vi "SubVI PhaseSpace.vi"() -> ()   [LabVIEW 2011]
uses:
  NCML-PhaseSpace/ctrOWLMarker.ctl
  ctlSeqFNs_SubVI PhaseSpace.ctl
  ctlPkgPhaseSpace.ctl
  ctlSeqFNs_SubVI ATI.ctl
  ctlTrialState.ctl
  ctlSeqFNs.ctl
  NCML-PhaseSpace/ctrCommonFlags.ctl
  NCML-PhaseSpace/ctrSetsFlags.ctl
  GLOBAL -MAIN.vi
  C:/Program Files/Phasespace/libowlsock.dll
panel:
  out "Hz":dbl(graph)
  out "save file":path
  in  "Read Cycle Time (s)":dbl=0.05 min=0.01 max=10.0 step=0.01 format="%.2f"
  out "recording?":bool
  out "markers obtained (err: <0)":u16
  out "markers":T1[](array[typedef])
  in  "marker count":i32=16
  out "connected?":bool
  in  "server IP":string="192.168.0.101"
  in  "STOP":bool
  # "Parallel SubVI PhaseSpace"
  # "Acquires PhaseSpace data and Trigger signal\nSaves TDMS file."
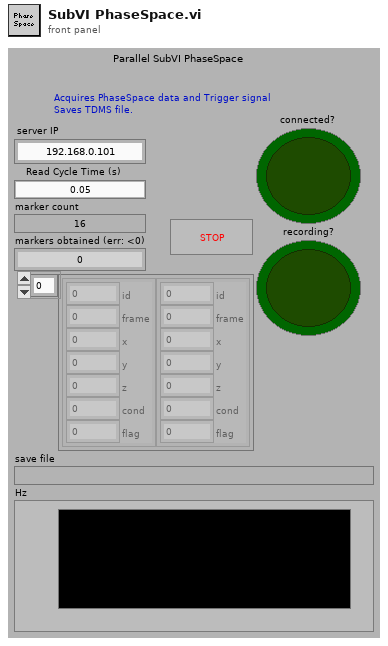
[diagram p1: front panel]
types:
  T1 = typedef "ctrOWLMarker.ctl" = cluster{"id":i32, "frame":i32, "x":sgl, "y":sgl, "z":sgl, "cond":sgl, "flag":u32}
  T2 = typedef "ctlPkgPhaseSpace.ctl" = cluster{"VIRef":refnum<vi>, "PhaseSpace":refnum<k34>, "PhaseSpace Ch names":string[], "Markers":T1[], "Markers Ch count":i32, "tick ini":i64, "ATI":refnum<queue>, "Trigger events":T3, "connected to server?":bool, "recording?":bool, "MAIN":refnum<queue>, "tick pre":i64, "Markers count":u16}
  T3 = typedef "ctlTrialState.ctl" = enum16{"no events", "ready", "start", "hold", "stop", "end"}
  T4 = typedef "ctlSeqFNs_SubVI PhaseSpace.ctl" = enum16{"INITIALIZE", "IDLE", "READY", "SEND2MAIN", "TRIGGER", "END", "ERROR", "EXIT"}
  T5 = typedef "ctlSeqFNs.ctl" = enum16{"INITIALIZE MAIN", "UpdateProtocol", "INITIALIZE Sub", "IDLE", "Ready", "Events", "Get PhaseSpace", "Get ATI", "Finish", "End PhaseSpace", "End ATI", "ERROR", "EXIT"}
  T6 = typedef "ctlSeqFNs_SubVI ATI.ctl" = enum16{"INITIALIZE", "IDLE", "READY", "SEND2MAIN", "CALIB Load", "BIAS", "TRIGGER", "END", "ERROR", "EXIT"}
  T7 = enum16{"ALIGN -CENTER", "ALIGN -TOP LEFT", "ALIGN -AS IS", "ALIGN -CUSTOM"}
  T8 = typedef "ctrCommonFlags.ctl" = u16
  T9 = typedef "ctrSetsFlags.ctl" = u16
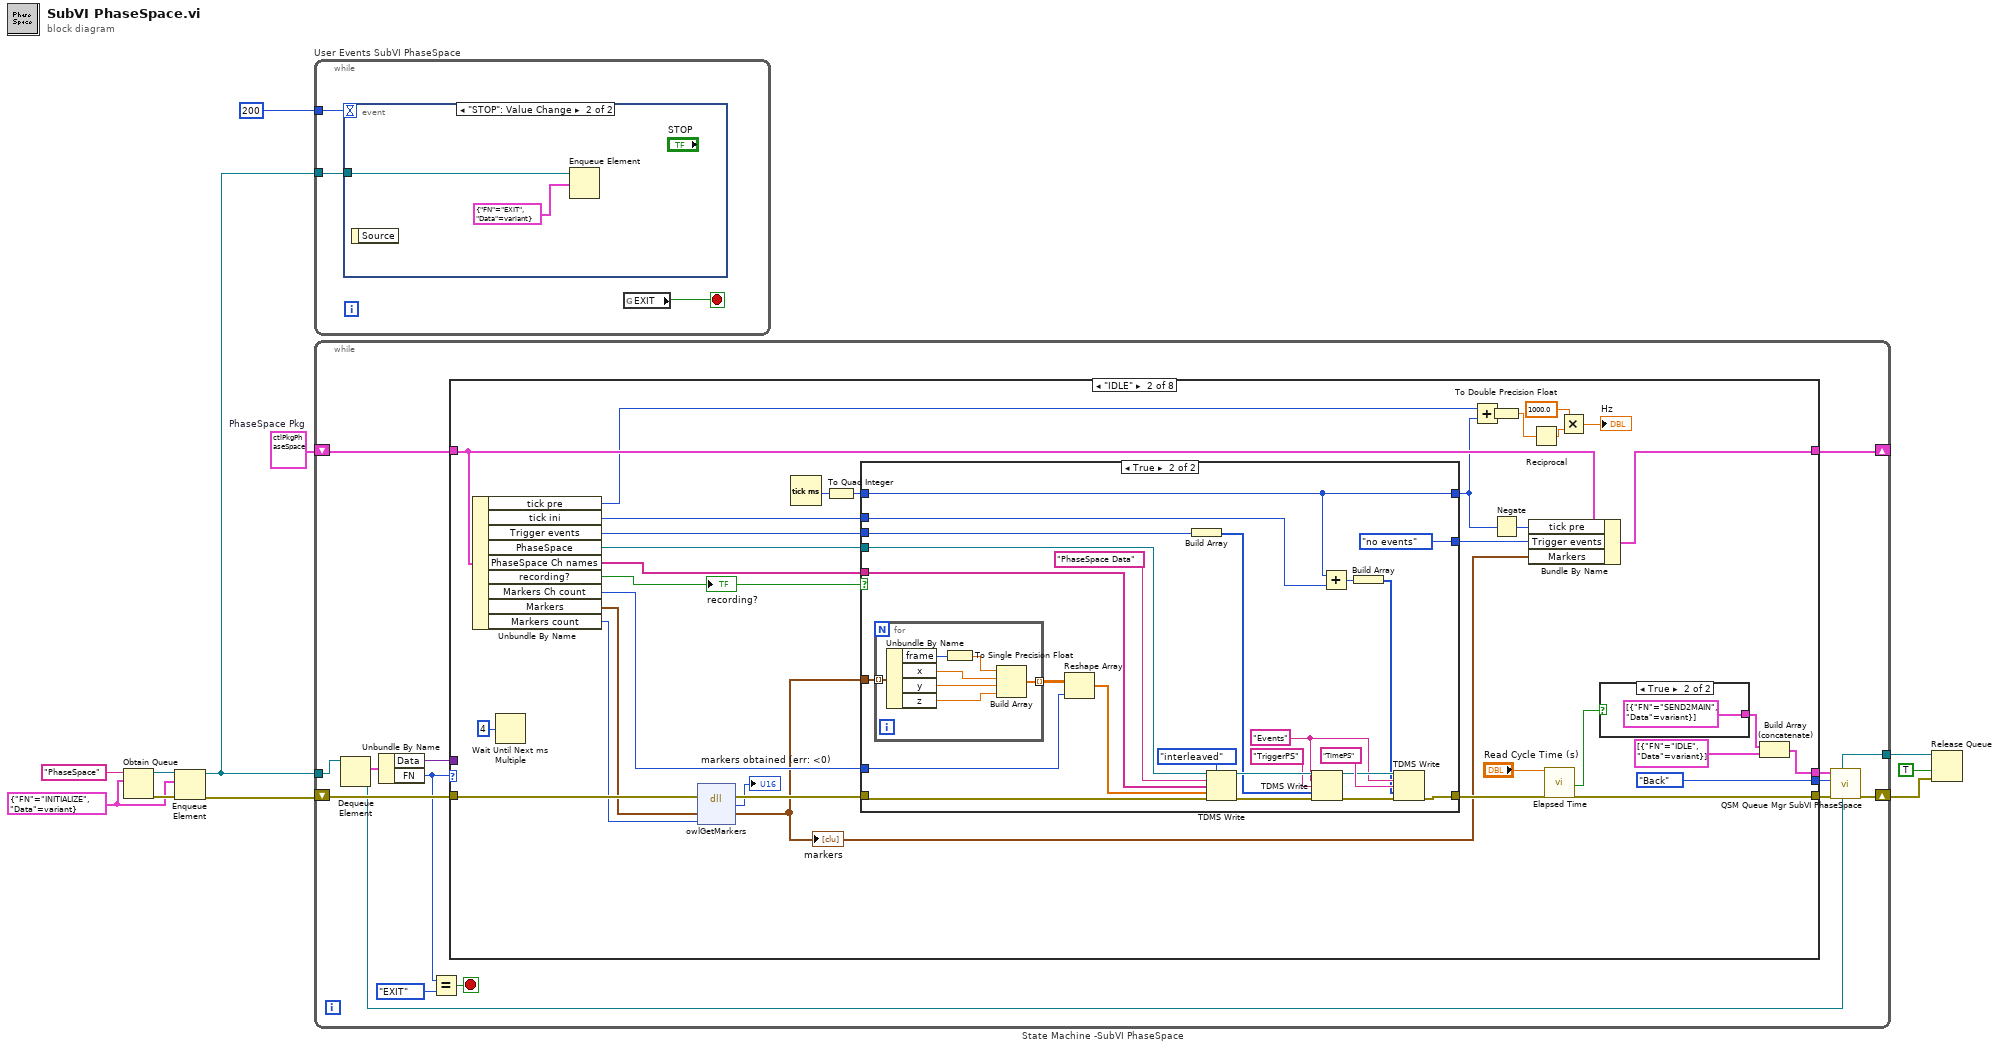
[diagram p0: block diagram]
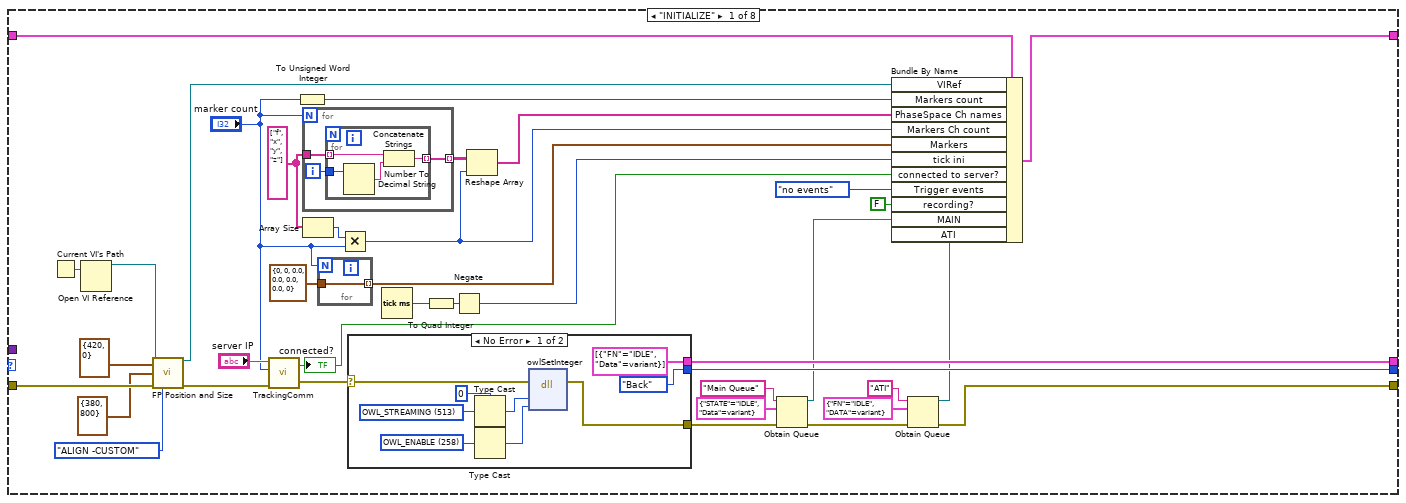
[diagram p2: hidden frame]
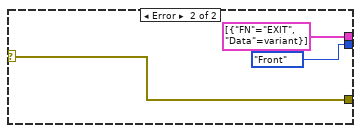
[diagram p3: hidden frame]
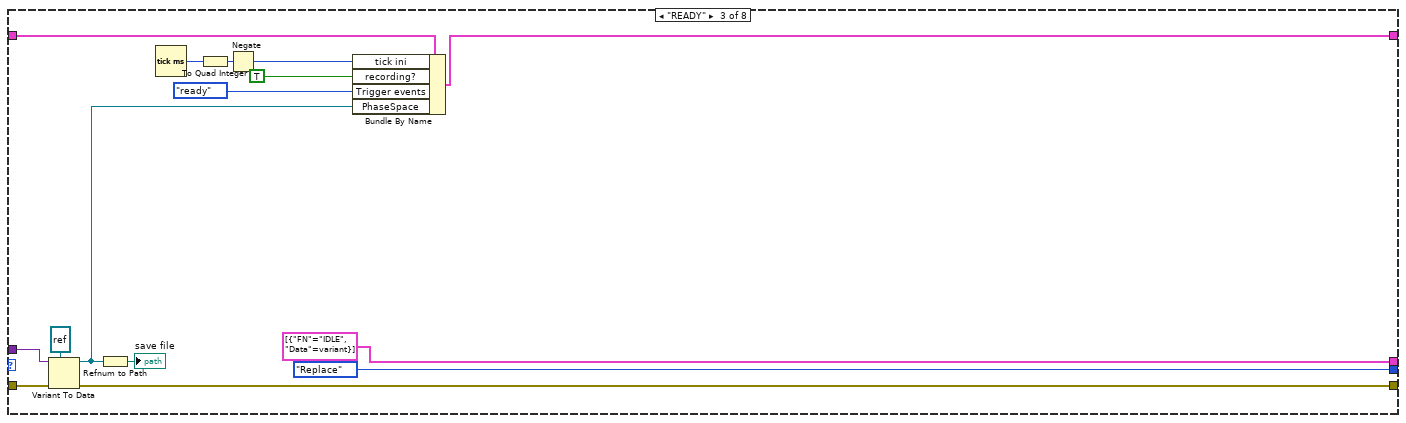
[diagram p6: hidden frame]
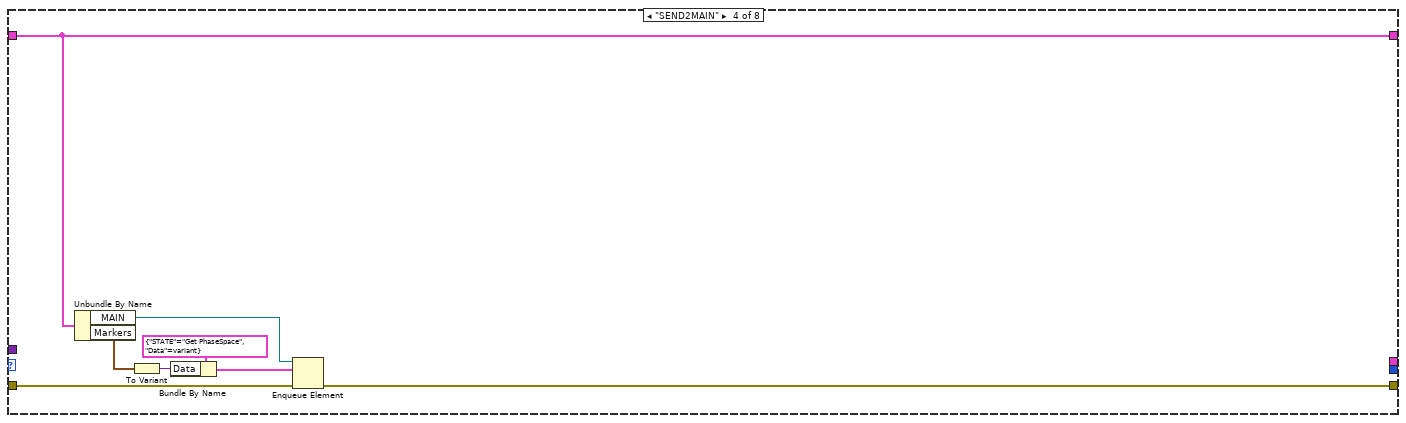
[diagram p7: hidden frame]
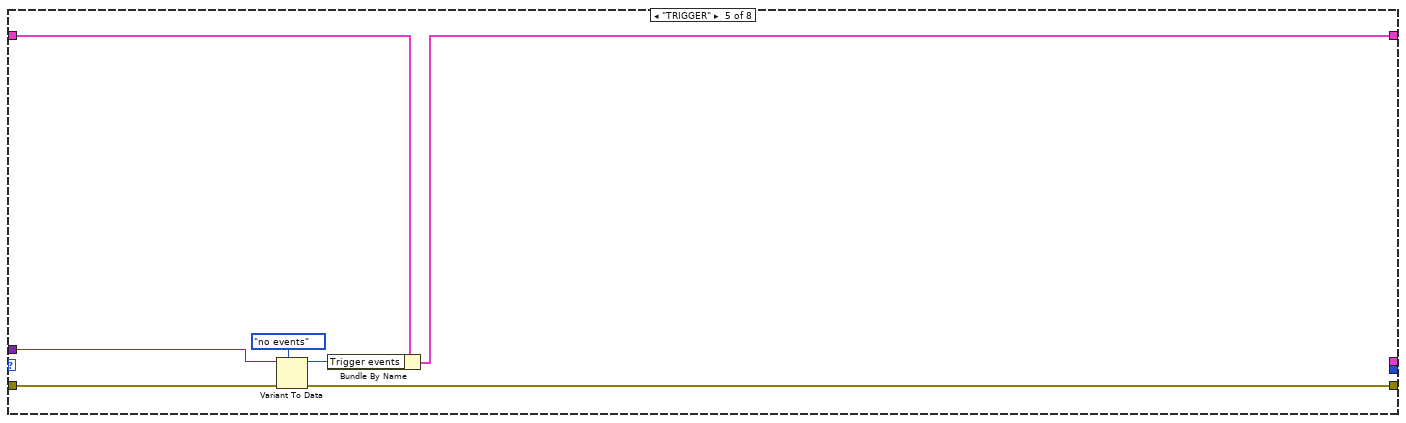
[diagram p8: hidden frame]
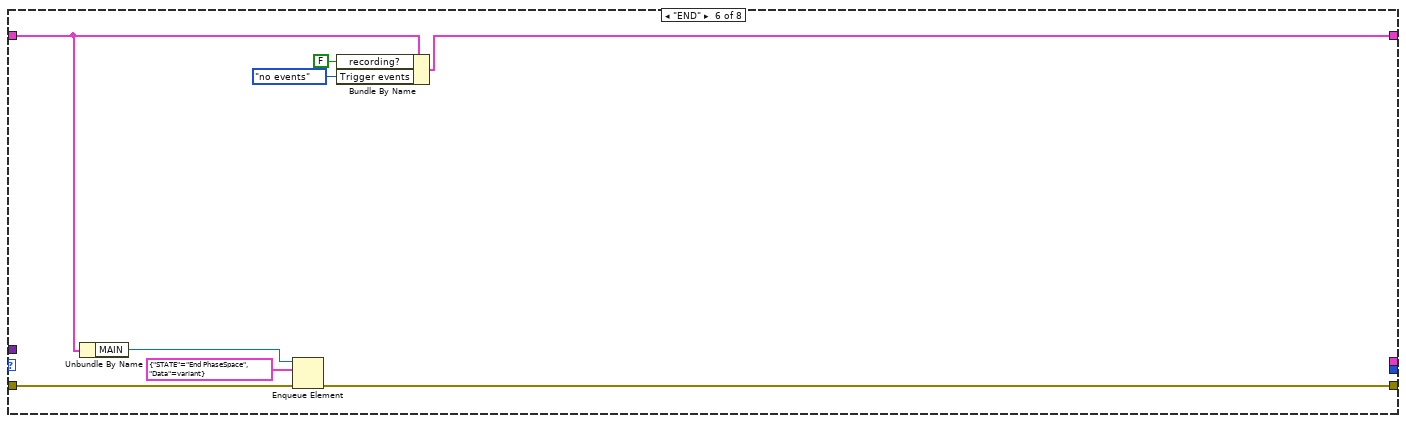
[diagram p9: hidden frame]
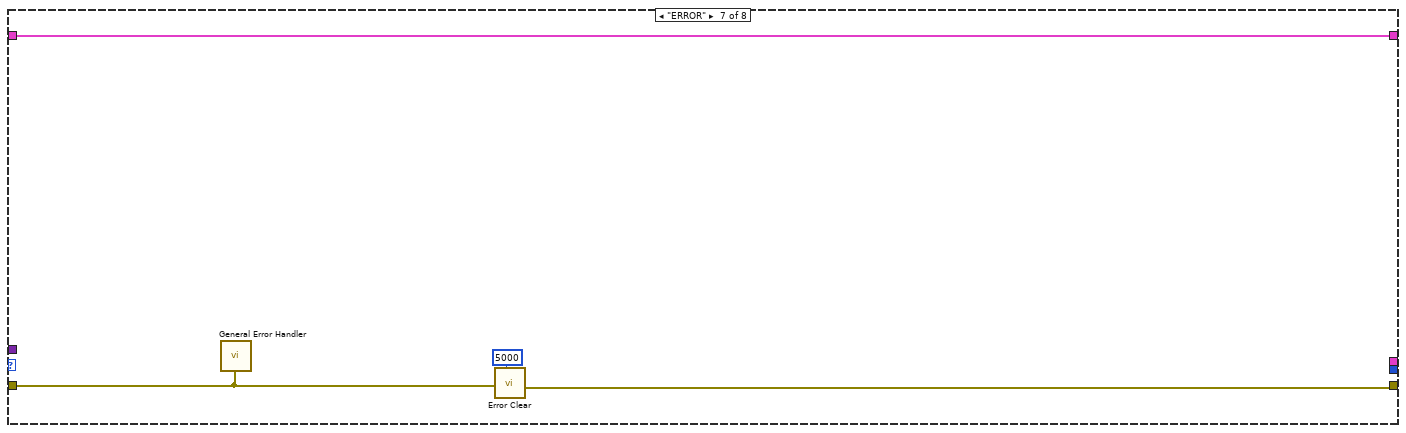
[diagram p10: hidden frame]
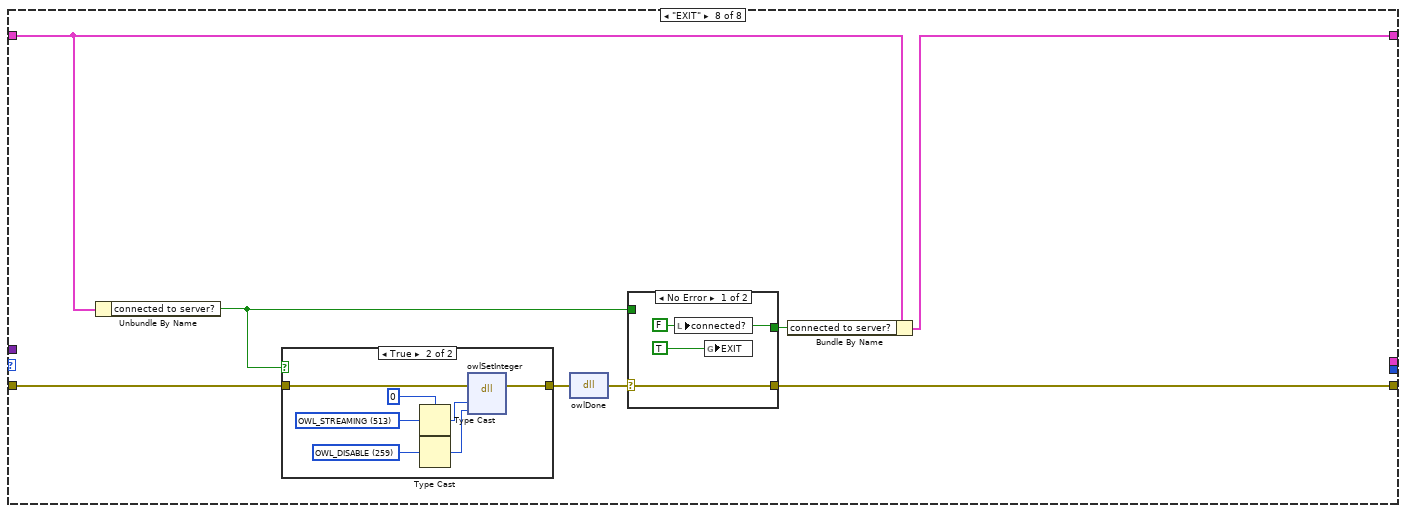
[diagram p11: hidden frame]
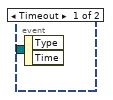
[diagram p14: hidden frame]
diagram:
  w2 = T2 {"VIRef"=refnum, "PhaseSpace"=refnum, "PhaseSpace Ch names"=[], "Markers"=[], "Markers Ch count"=0, "tick ini"=0, "ATI"=refnum, "Trigger events"=enum."no events", "connected to server?"=FALSE, "recording?"=FALSE, "MAIN"=refnum, "tick pre"=0, "Markers count"=0}  # PhaseSpace Pkg
  w6 = cluster{"FN":T4, "Data":variant} {"FN"=enum."INITIALIZE", "Data"=variant} ("cluFNData")
  n1 = Obtain Queue(name (unnamed)="PhaseSpace", element data type=w6) -> (queue out=w7:refnum<queue>, error out=w9:errorcluster)  [unwired: 3 in, 1 out]
  n2 = Enqueue Element(queue=w7, element=w6, error in (no error)=w9) -> (queue out=w3:refnum<queue>, error out=w8:errorcluster)  [unwired: 1 in, 1 out]
  n3 = while "User Events SubVI PhaseSpace" {
    tunnel: 200 -> [w14]
    tunnel: w3 -> [w12]
    stop <- w13 stop-if-true
    n4 = event shown="[1] \"STOP\": Value Change" {
      selector: _ -> [_ _]
      dyn-events: _ -> [_ _]
      timeout: w14 -> [_ _]
      tunnel: w12 -> [_ w16]
      event Timeout {
        n5 = event-data() -> ()  [unwired: 1 in, 2 out]
      }
      event "STOP": Value Change {
        n6 = event-data() -> ()  [unwired: 1 in, 1 out]
        n7 = Enqueue Element(queue=w16, element=cluster{"FN":T4, "Data":variant} {"FN"=enum."EXIT", "Data"=variant}) -> ()  [unwired: 2 in, 3 out]
      }
    }
    n8 = global read "GLOBAL -MAIN.vi" "EXIT"() -> (w13:bool)
  }
  n9 = while "State Machine -SubVI PhaseSpace" {
    shift-right: [w20] -> w1
    shift-left: w8 -> [w30]
    tunnel: w3 -> [w27]
    tunnel: [w17] -> w5
    shift-right: [w22] -> _
    shift-left: w2 -> [w23]
    stop <- w29 stop-if-true
    n10 = Dequeue Element(queue=w27) -> (queue out=w17:refnum<queue>, element=w26:cluster{"FN":T4, "Data":variant})  [unwired: 2 in, 2 out]
    n11 = Unbundle By Name(w26) -> ("Data"=w25:variant, "FN"=w24:T4)
    n12 = Equal?(x=w24, y=ctlSeqFNs_SubVI_PhaseSpace."EXIT" ("FN")) -> (x = y?=w29:bool)
    n13 = case shown="\"IDLE\"" w24 {
      tunnel: w30 -> [w66 w118 w163 w180 w187 w188 w196 w200]
      tunnel: [w61 w108 w162 w179 w186 w189 w198 w201] -> w21
      tunnel: w25 -> [_ _ w164 _ w185 _ _ _]
      tunnel: w23 -> [w48 w107 w168 w178 w183 w190 w199 w206]
      tunnel: [w65 w106 w172 w178 w184 w195 w199 w205] -> w22
      tunnel: [w43 w112 cluster{"FN":T4, "Data":variant}[] [{"FN"=enum."IDLE", "Data"=variant}] ("QFNs") _ _ _ _ _] -> w18
      tunnel: [w42 enum16{"Back", "Front", "Replace"}."Back" ("Enum") enum16{"Back", "Front", "Replace"}."Replace" ("Enum") _ _ _ _ _] -> w19
      frame "INITIALIZE" {
        w49 = string[] ["f", "x", "y", "z"]
        n14 = Current VI's Path() -> (path=w68:path)
        n15 = Open VI Reference(vi path=w68) -> (vi reference=w67:refnum<vi>)  [unwired: 5 in, 1 out]
        n16 = call "FP Position and Size.vi"("VIRefNum  IN"=w67, "Poistion"=cluster{"left":i16, "top":i16} {"left"=420, "top"=0}, "Size"=cluster{"right":i16, "bottom":i16} {"right"=380, "bottom"=800}, "error in (no error)"=w66, "Mode"=T7."ALIGN -CUSTOM") -> ("VIRefNum OUT"=w33:refnum<vi>, "error out"=w55:errorcluster)  [unwired: 9 in]
        n17 = call "TrackingComm.vi"("error in (no error)"=w55, "marker tally (default: 32)"="marker count", "server address"="server IP") -> ("error out"=w56:errorcluster, "connected to server?"=w40:bool)  [unwired: 1 in]
        "connected?" <- w40
        n18 = To Unsigned Word Integer(number="marker count") -> (unsigned 16bit integer=w31:u16)
        n19 = for {
          N: "marker count" -> [_]
          tunnel: w49 -> [w71]
          tunnel: [w69] -> w53 mode=indexing
          i -> [w70]
          n20 = for {
            tunnel: w71 -> [w75] mode=indexing
            tunnel: w70 -> [w74]
            tunnel: [w72] -> w69 mode=indexing
            n21 = Number To Decimal String(number=w74) -> (decimal integer string=w73:string)  [unwired: 1 in]
            n22 = Concatenate Strings(w75, w73) -> (w72:string)
          }
        }
        n23 = Array Size(array=w49) -> (size(s)=w50:i32)
        n24 = for {
          N: "marker count" -> [_]
          tunnel: T1 {"id"=0, "frame"=0, "x"=0.0, "y"=0.0, "z"=0.0, "cond"=0.0, "flag"=0} -> [w88]
          tunnel: [w88] -> w45 mode=indexing
        }
        n25 = Multiply(x=w50, y="marker count") -> (x*y=w44:i32)
        n26 = case shown="No Error" w56 {
          selector: w56 -> [w79 w87]
          tunnel: [w78 w87] -> w54
          tunnel: [cluster{"FN":T4, "Data":variant}[] [{"FN"=enum."IDLE", "Data"=variant}] ("QFNs") cluster{"FN":T4, "Data":variant}[] [{"FN"=enum."EXIT", "Data"=variant}] ("QFNs")] -> w43
          tunnel: [enum16{"Back", "Front", "Replace"}."Back" ("Enum") enum16{"Back", "Front", "Replace"}."Front" ("Enum")] -> w42
          frame No Error {
            w84 = u16 0
            w81 = T8 258 items=["OWL_CREATE"=256, "OWL_DESTROY"=257, "OWL_ENABLE"=258, "OWL_DISABLE"=259] ("Common flages")
            w80 = T9 513 items=["OWL_FREQUENCY"=512, "OWL_STREAMING"=513, "OWL_INTERPOLATION"=514, "OWL_BUTTONS"=528, "OWL_MARKERS"=529, "OWL_RIGIDS"=530, "OWL_COMMDATA"=544, "OWL_TIMESTAMP"=545, "OWL_PLANES"=672, "OWL_DETECTORS"=673, "OWL_IMAGES"=674, "OWL_TRANSFORM"=49664] ("Sets flags")
            n27 = Type Cast(type=w84, x=w80) -> (*(type *) &x=w83:u16)
            n28 = Type Cast(type=w84, x=w81) -> (*(type *) &x=w82:u16)
            n29 = dll-call lib="C:/Program Files/Phasespace/libowlsock.dll" fn="owlSetInteger"(error in=w79, "pname"=w83, "param"=w82) -> (error out=w78:errorcluster)  [unwired: 4 in, 2 out]
          }
          frame Error {
          }
        }
        n30 = Tick Count (ms)() -> (millisecond timer value=w51:u32)
        n31 = To Quad Integer(1:w51) -> (0:w52:i64)
        n32 = Negate(x=w52) -> (-x=w47:i64)
        n33 = Reshape Array(w53, w44) -> (w46:string[])
        n34 = Obtain Queue(name (unnamed)="Main Queue", element data type=cluster{"STATE":T5, "Data":variant} {"STATE"=enum."IDLE", "Data"=variant} ("element"), error in (no error)=w54) -> (queue out=w35:refnum<queue>, error out=w39:errorcluster)  [unwired: 2 in, 1 out]
        n35 = Obtain Queue(name (unnamed)="ATI", element data type=cluster{"FN":T6, "DATA":variant} {"FN"=enum."IDLE", "DATA"=variant} ("cluFNData"), error in (no error)=w39) -> (queue out=w36:refnum<queue>, error out=w61:errorcluster)  [unwired: 2 in, 1 out]
        n36 = Bundle By Name(cluster=w48, "VIRef"=w33, "Markers count"=w31, "PhaseSpace Ch names"=w46, "Markers Ch count"=w44, "Markers"=w45, "tick ini"=w47, "connected to server?"=w40, "Trigger events"=ctlTrialState."no events", "recording?"=FALSE, "MAIN"=w35, "ATI"=w36) -> (w65:T2)
      }
      frame "IDLE" {
        n37 = Unbundle By Name(w107) -> ("tick pre"=w101:i64, "tick ini"=w103:i64, "Trigger events"=w115:T3, "PhaseSpace"=w120:refnum<k34>, "PhaseSpace Ch names"=w121:string[], "recording?"=w114:bool, "Markers Ch count"=w102:i32, "Markers"=w104:T1[], "Markers count"=w93:u16)
        "recording?" <- w114
        n38 = Wait Until Next ms Multiple(millisecond multiple=u32 4) -> ()  [unwired: 1 out]
        n39 = dll-call lib="C:/Program Files/Phasespace/libowlsock.dll" fn="owlGetMarkers"(error in=w118, "markers"=w104, "count"=w93) -> (error out=w119:errorcluster, "return type"=→"markers obtained (err: <0)":u16, "markers"=w89:T1[])  [unwired: 3 in, 1 out]
        "markers" <- w89
        n40 = Tick Count (ms)() -> (millisecond timer value=w92:u32)
        n41 = To Quad Integer(1:w92) -> (0:w91:i64)
        n42 = case shown="True" w114 {
          tunnel: w121 -> [_ w148]
          tunnel: w120 -> [_ w147]
          tunnel: w119 -> [w126 w146]
          tunnel: [w126 w144] -> w109
          tunnel: w115 -> [w125 w137]
          tunnel: [w125 ctlTrialState."no events" ("Trigger events")] -> w105
          tunnel: w103 -> [_ w127]
          tunnel: w102 -> [_ w132]
          tunnel: w89 -> [_ w131]
          tunnel: [w124 w128] -> w100
          tunnel: w91 -> [w124 w128]
          frame False {
          }
          frame True {
            w139 = "Events" ("group name")
            n43 = for {
              tunnel: w131 -> [w157] mode=indexing
              tunnel: [w153] -> w134 mode=indexing
              n44 = Unbundle By Name(w157) -> ("frame"=w152:i32, "x"=w156:sgl, "y"=w155:sgl, "z"=w154:sgl)
              n45 = To Single Precision Float(number=w152) -> (single precision float=w151:sgl)
              n46 = Build Array(w151, w156, w155, w154) -> (w153:sgl[])
            }
            n47 = Reshape Array(w134, w132) -> (w133:sgl[])
            n48 = Build Array(w137) -> (w130:T3[])
            n49 = TDMS Write(0:w147, 1:enum16{"decimated", "interleaved"}."interleaved" ("data layout (0:decimated)"), 5:"PhaseSpace Data" ("group name"), 7:w148, 9:w133, 11:w146) -> (4:w143:refnum<k34>, 15:w142:errorcluster)  [unwired: 2 out]
            n50 = TDMS Write(0:w143, 5:w139, 7:"TriggerPS" ("channel name"), 9:w130, 11:w142) -> (4:w140:refnum<k34>, 15:w141:errorcluster)  [unwired: 1 in, 2 out]
            n51 = Add(x=w128, y=w127) -> (x+y=w136:i64)
            n52 = Build Array(w136) -> (w135:i64[])
            n53 = TDMS Write(0:w140, 5:w139, 7:"TimePS" ("channel name"), 9:w135, 11:w141) -> (15:w144:errorcluster)  [unwired: 1 in, 3 out]
          }
        }
        n54 = Add(x=w101, y=w100) -> (x+y=w97:i64)
        n55 = To Double Precision Float(number=w97) -> (double precision float=w96:dbl)
        n56 = Negate(x=w100) -> (-x=w90:i64)
        n57 = Bundle By Name(cluster=w107, "tick pre"=w90, "Trigger events"=w105, "Markers"=w89) -> (w106:T2)
        n58 = Reciprocal(x=w96) -> (1/x=w98:dbl)
        n59 = call "Elapsed Time"("Time Target (s)"="Read Cycle Time (s)", "error in (no error)"=w109) -> ("Time has Elapsed"=w110:bool, "error out"=w108:errorcluster)  [unwired: 10 in, 6 out]
        n60 = Multiply(x=1000.0, y=w98) -> (x*y=→"Hz":dbl)
        n61 = case shown="True" w110 {
          tunnel: [_ cluster{"FN":T4, "Data":variant}[] [{"FN"=enum."SEND2MAIN", "Data"=variant}] ("QFNs")] -> w111
          frame False {
          }
          frame True {
          }
        }
        n62 = Build Array (concatenate)(w111, cluster{"FN":T4, "Data":variant}[] [{"FN"=enum."IDLE", "Data"=variant}] ("QFNs")) -> (w112:cluster{"FN":T4, "Data":variant}[])
      }
      frame "READY" {
        n63 = Variant To Data(error in=w163, type=refnum<k34> refnum ("tdms file out"), Variant=w164) -> (data=w161:refnum<k34>, error out=w162:errorcluster)
        n64 = Refnum to Path(1:w161) -> (0:→"save file":path)
        n65 = Tick Count (ms)() -> (millisecond timer value=w167:u32)
        n66 = To Quad Integer(1:w167) -> (0:w166:i64)
        n67 = Negate(x=w166) -> (-x=w165:i64)
        n68 = Bundle By Name(cluster=w168, "tick ini"=w165, "recording?"=TRUE, "Trigger events"=ctlTrialState."ready", "PhaseSpace"=w161) -> (w172:T2)
      }
      frame "SEND2MAIN" {
        n69 = Unbundle By Name(w178) -> ("MAIN"=w177:refnum<queue>, "Markers"=w176:T1[])
        n70 = To Variant(anything=w176) -> (Variant=w175:variant)
        n71 = Bundle By Name(cluster=cluster{"STATE":T5, "Data":variant} {"STATE"=enum."Get PhaseSpace", "Data"=variant} ("element"), "Data"=w175) -> (w173:cluster{"STATE":T5, "Data":variant})
        n72 = Enqueue Element(queue=w177, element=w173, error in (no error)=w180) -> (error out=w179:errorcluster)  [unwired: 1 in, 2 out]
      }
      frame "TRIGGER" {
        n73 = Variant To Data(error in=w187, type=ctlTrialState."no events" ("Trigger events"), Variant=w185) -> (data=w181:T3, error out=w186:errorcluster)
        n74 = Bundle By Name(cluster=w183, "Trigger events"=w181) -> (w184:T2)
      }
      frame "END" {
        n75 = Unbundle By Name(w190) -> ("MAIN"=w192:refnum<queue>)
        n76 = Enqueue Element(queue=w192, element=cluster{"STATE":T5, "Data":variant} {"STATE"=enum."End PhaseSpace", "Data"=variant}, error in (no error)=w188) -> (error out=w189:errorcluster)  [unwired: 1 in, 2 out]
        n77 = Bundle By Name(cluster=w190, "recording?"=FALSE, "Trigger events"=ctlTrialState."no events") -> (w195:T2)
      }
      frame "ERROR" {
        n78 = call <vilib>:"General Error Handler.vi"("error in (no error)"=w196) -> ()  [unwired: 10 in, 5 out]
        n79 = call "Error Clear.vi"("wait(ms)"=u32 5000, "error in"=w196) -> ("error in (no error)"=w198:errorcluster)  [unwired: 6 in]
      }
      frame "EXIT" {
        n80 = Unbundle By Name(w206) -> ("connected to server?"=w202:bool)
        n81 = case shown="True" w202 {
          tunnel: w200 -> [w213 w215]
          tunnel: [w213 w214] -> w207
          frame False {
          }
          frame True {
            w218 = u16 0
            w217 = T8 259 items=["OWL_CREATE"=256, "OWL_DESTROY"=257, "OWL_ENABLE"=258, "OWL_DISABLE"=259] ("Common flages")
            w216 = T9 513 items=["OWL_FREQUENCY"=512, "OWL_STREAMING"=513, "OWL_INTERPOLATION"=514, "OWL_BUTTONS"=528, "OWL_MARKERS"=529, "OWL_RIGIDS"=530, "OWL_COMMDATA"=544, "OWL_TIMESTAMP"=545, "OWL_PLANES"=672, "OWL_DETECTORS"=673, "OWL_IMAGES"=674, "OWL_TRANSFORM"=49664] ("Sets flags")
            n82 = Type Cast(type=w218, x=w216) -> (*(type *) &x=w219:u16)
            n83 = Type Cast(type=w218, x=w217) -> (*(type *) &x=w220:u16)
            n84 = dll-call lib="C:/Program Files/Phasespace/libowlsock.dll" fn="owlSetInteger"(error in=w215, "pname"=w219, "param"=w220) -> (error out=w214:errorcluster)  [unwired: 4 in, 2 out]
          }
        }
        n85 = dll-call lib="C:/Program Files/Phasespace/libowlsock.dll" fn="owlDone"(error in=w207) -> (error out=w204:errorcluster)  [unwired: 2 in, 2 out]
        n86 = case shown="No Error" w204 {
          selector: w204 -> [w208 w211]
          tunnel: [w210 w212] -> w203
          tunnel: w202 -> [_ w212]
          tunnel: [w208 w211] -> w201
          frame No Error {
            w210 = FALSE ("connected to server?")
            n87 = local write "connected?"(w210) -> ()
            n88 = global write "GLOBAL -MAIN.vi" "EXIT"(TRUE ("EXIT")) -> ()
          }
          frame Error {
          }
        }
        n89 = Bundle By Name(cluster=w206, "connected to server?"=w203) -> (w205:T2)
      }
    }
    n90 = call "QSM Queue Mgr SubVI PhaseSpace.vi"("QRef"=w17, "Error IN"=w21, "FNs"=w19, "QSTATES"=w18) -> ("Error OUT"=w20:errorcluster)  [unwired: 4 in]
  }
  n91 = Release Queue(queue=w5, force destroy? (F)=TRUE, error in (no error)=w1) -> ()  [unwired: 3 out]
